vi "RIGOL DG4000 Series Frequency Sweep.vi"() -> ()   [LabVIEW 2012]
doc: "This example shows how to configure and enable a frequency sweep."
uses:
  <instrlib>/RIGOL DG4000 Series/Public/Configure/Configure Waveform Characteristics(Amplitude).vi
  <instrlib>/RIGOL DG4000 Series/Public/Configure/Configure Waveform Characteristics(Shape).vi
  <instrlib>/RIGOL DG4000 Series/RIGOL DG4000 Series.lvlib
panel:
  in  "Waveform Shape (0: Sinusoid)":i32(ring) items=["Sinusoid", "Square", "Ramp", "Pulse", "Noise", "User", "Harmonic", "Custom", "DC", "AbsSine", "AbsSineHalf", "AmpALT", "AttALT", "GaussPulse", "NegRamp", "NPulse", "PPulse", "SineTra", "SineVer", "StairDn", "StairUD", "StairUp", "Trapezia", "BandLimited", "Butterworth", "Chebyshev1", "Chebyshev2", "Combin", "CPulse", "CWPulse", "DampedOsc", "DualTone", "Gamma", "GateVibr", "LEMPulse", "MCNoise", "Discharge", "Pahcur", "Quake", "Radar", "Ripple", "RoundHalf", "RoundPM", "StepResp", "SwingOsc", "TV", "Voice", "AM", "FM", "PM", "PWM", "PFM", "Cardiac", "EOG", "EEG", "EMG", "Pulseilogram", "ResSpeed", "LFPulse", "Tens1", "Tens2", "Tens3", "Lgnition", "ISO16750-2 SP", "ISO16750-2 VR", "ISO7637-2 TP1", "ISO7637-2 TP2A", "ISO7637-2 TP2B", "ISO7637-2 TP3A", "ISO7637-2 TP3B", "ISO7637-2 TP4", "ISO7637-2 TP5A", "ISO7637-2 TP5B", "SCR", "Surge", "Airy", "Besselj", "Bessely", "Cauchy", "Cubic", "Dirichlet", "Erf", "Erfc", "Erfclnv", "Erflnv", "ExpFall", "ExpRise", "Gauss", "HaverSine", "Laguerre", "Laplace", "Legend", "Log", "LogNormal", "Lorentz", "Maxwell", "Rayleigh", "Versiera", "Weibull", "ARB_X2", "CosH", "CosInt", "Cot", "CotHCon", "CotHPro", "CscCon", "CscPro", "CscHCon", "CscHPro", "RecipCon", "RecipPro", "SecCon", "SecPro", "SecH", "Sinc", "SinH", "SinInt", "Sqrt", "Tan", "TanH", "ACos", "ACosH", "ACotCon", "ACotPro", "ACotHCon", "ACotHPro", "ACscCon", "ACscPro", "ACscHCon", "ACscHPro", "ASecCon", "ASsePro", "ASecH", "ASin", "ASinH", "ATan", "ATanH", "Barlett", "BarthannWin", "Blackman", "BlackmanH", "BlackmanWin", "Boxcar", "ChebWin", "FlattopWin", "Hamming", "Hanning", "Kaiser", "NuttallWin", "ParzenWin", "TaylorWin", "Triang", "TukeyWin"]
  in  "Output Channel (1: Channel 1)":i32(ring)=1 items=["Channel 1"=1, "Channel 2"=2]
  in  "Sweep Time (1.00 s)":dbl=1.0 format="%#.6g"
  in  "Stop  Frequency  (1000.0 Hz)":dbl=1000.0 format="%#.6g"
  in  "Start Frequency (100.0 Hz)":dbl=100.0 format="%#.6g"
  in  "Amplitude (0.1 Vpp)":dbl=0.1
  in  "VISA resource name":refnum<visa-resource-name>
  # "(c) 2012 National Instruments.  ALL RIGHTS RESERVED."
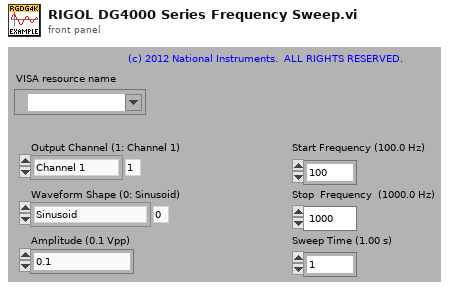
[diagram p1: front panel]
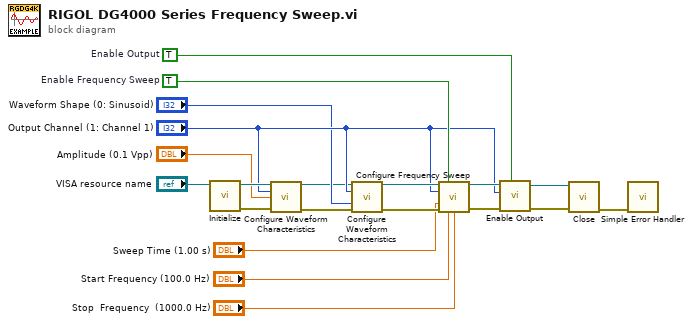
[diagram p0: block diagram]
diagram:
  w13 = TRUE  # Enable Output
  w10 = TRUE  # Enable Frequency Sweep
  n1 = call <instrlib>:"Initialize.vi"("VISA resource name"="VISA resource name") -> ("error out"=w6:errorcluster, "VISA resource name out"=w7:refnum<visa-resource-name>)  [unwired: 4 in, 5 out]
  n2 = call-poly <instrlib>:"Configure Waveform Characteristics.vi"("VISA resource name"=w7, "Output Channel (1: Channel 1)"="Output Channel (1: Channel 1)", "Amplitude (5)"="Amplitude (0.1 Vpp)", "error in (no error)"=w6) -> ("VISA resource name out"=w2:refnum<visa-resource-name>, "error out"=w1:errorcluster)  [unwired: 4 in, 6 out]
  n3 = call-poly <instrlib>:"Configure Waveform Characteristics.vi"("VISA resource name"=w2, "Output Channel (1: Channel 1)"="Output Channel (1: Channel 1)", "Waveform Shape (0: Sinusoid)"="Waveform Shape (0: Sinusoid)", "error in (no error)"=w1) -> ("VISA resource name out"=w12:refnum<visa-resource-name>, "error out"=w11:errorcluster)  [unwired: 10 out]
  n4 = call <instrlib>:"Configure Frequency Sweep.vi"("VISA resource name"=w12, "Enable Frequency Sweep (T: Enable)"=w10, "Output Channel (1: Channel 1)"="Output Channel (1: Channel 1)", "Sweep Time (1 s)"="Sweep Time (1.00 s)", "error in (no error)"=w11, "Start Frequency (100 Hz)"="Start Frequency (100.0 Hz)", "Stop Frequency (1000 Hz)"="Stop  Frequency  (1000.0 Hz)") -> ("VISA resource name out"=w17:refnum<visa-resource-name>, "error out"=w16:errorcluster)  [unwired: 2 in, 5 out]
  n5 = call <instrlib>:"Enable Output.vi"("Enable Output (T: Enable)"=w13, "error in (no error)"=w16, "Output Channel (1: Channel 1)"="Output Channel (1: Channel 1)", "VISA resource name"=w17) -> ("error out"=w15:errorcluster, "VISA resource name out"=w14:refnum<visa-resource-name>)  [unwired: 6 out]
  n6 = call <instrlib>:"Close.vi"("error in (no error)"=w15, "VISA resource name"=w14) -> ("error out"=w20:errorcluster)  [unwired: 9 out]
  n7 = call <vilib>:"Simple Error Handler.vi"("error in (no error)"=w20) -> ()  [unwired: 1 in, 8 out]
